vi "Teleop.vi"(10 "Match Info":T1={"Autonomous Elapsed Seconds"=0.0, "TeleOp Elapsed Seconds"=0.0, "Disabled Elapsed Seconds"=0.0, "Visited Autonomous"=FALSE, "Visited TeleOp"=FALSE, "Visited Disabled"=FALSE, "Autonomous Settings"={"Autonomous Style"=enum."Independent", "VI Refnum"=refnum}}, 11 "Call Context":T2) -> ()   [LabVIEW 2012]
doc: "This VI is called for each TeleOp packet received from the DS where the robot is not disabled. It is often used to read from the joysticks and update I/O or to update setpoints for timed control loops. It should complete and return within 20 milliseconds or it may miss DS packets."
uses:
  <vilib>/Rock Robotics/WPI/DriverStation/WPI_DriverStationDerivedRobotMode.ctl
  <vilib>/Rock Robotics/WPI/DriverStation/WPI_DriverStationMatch Info.ctl
  Global 1.vi
  Robot Global Data.vi
panel:
  in  "Boolean":bool
  in  "Percent":dbl
  out "RPM Number":dbl
  in  "RPM?":bool
  out "Actual RPM":dbl(slide) scale=0.0..4000.0
  in  "Input":dbl(slide) scale=0.0..1.0
  # "RPM"
  # "RPM"
  # "Power"
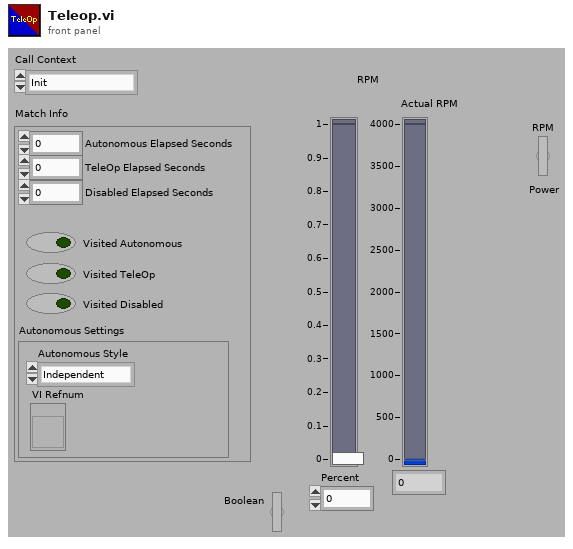
[diagram p1: front panel]
types:
  T1 = typedef "WPI_DriverStationMatch Info.ctl" = cluster{"Autonomous Elapsed Seconds":dbl, "TeleOp Elapsed Seconds":dbl, "Disabled Elapsed Seconds":dbl, "Visited Autonomous":bool, "Visited TeleOp":bool, "Visited Disabled":bool, "Autonomous Settings":cluster{"Autonomous Style":enum16{"Iterative", "Independent"}, "VI Refnum":refnum<vi>}}
  T2 = typedef "WPI_DriverStationDerivedRobotMode.ctl" = enum16{"Init", "Execute", "Stop"}
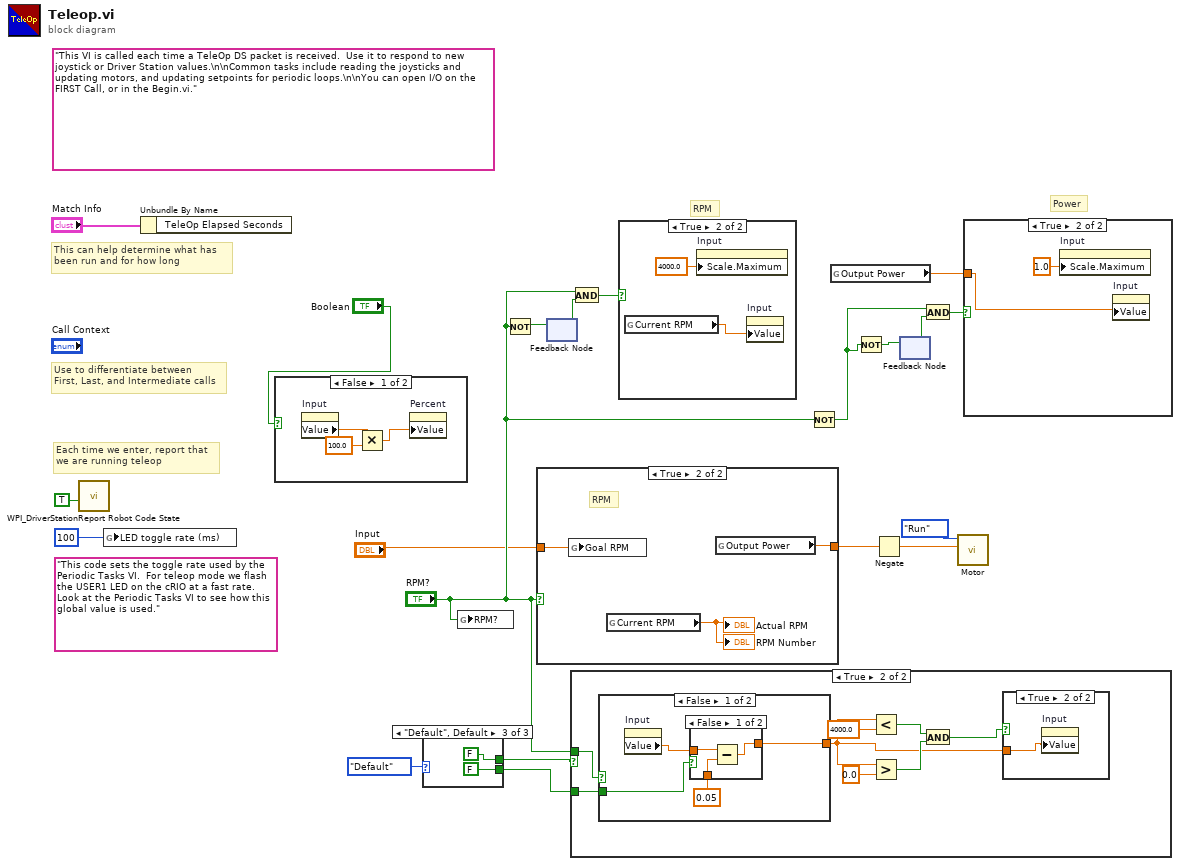
[diagram p0: block diagram]
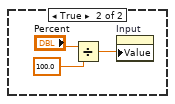
[diagram p2: hidden frame]
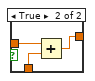
[diagram p5: hidden frame]
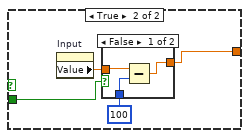
[diagram p6: hidden frame]
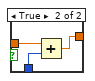
[diagram p7: hidden frame]
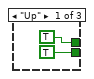
[diagram p8: hidden frame]
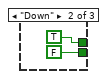
[diagram p9: hidden frame]
diagram:
  (unwired) "This code sets the toggle rate used by the Periodic Tasks VI.  For teleop mode we flash the USER1 LED on the cRIO at a fast rate.  Look at the Periodic Tasks VI to see how this global value is used."
  (unwired) "This VI is called each time a TeleOp DS packet is received.  Use it to respond to new joystick or Driver Station values.\n\nCommon tasks include reading the joysticks and updating motors, and updating setpoints for periodic loops.\n\nYou can open I/O on the FIRST Call, or in the Begin.vi."
  # "Power"
  # "RPM"
  # "Each time we enter, report that\nwe are running teleop"
  # "Use to differentiate between\nFirst, Last, and Intermediate calls"
  # "This can help determine what has\nbeen run and for how long"
  n1 = call <vilib>:"WPI_DriverStationReport Robot Code State.vi"("TeleOp"=TRUE ("Autonomous")) -> ()  [unwired: 10 in, 1 out]
  n2 = global write "Robot Global Data.vi" "LED toggle rate (ms)"(u32 100 ("LED ms toggle rate")) -> ()
  n3 = Unbundle By Name("Match Info") -> ()  [unwired: 1 out]
  n4 = case shown="False" "Boolean" {
    frame False {
      n5 = property on="Input" class="Slide (strict)"() -> ("Value"=w23:dbl)  [unwired: 2 in, 2 out]
      n6 = Multiply(x=w23, y=100.0) -> (x*y=w21:dbl)
      n7 = property on="Percent" class="DigNum (strict)"("Value"=w21) -> ()  [unwired: 2 in, 2 out]
    }
    frame True {
      n8 = Divide(x="Percent", y=100.0) -> (x/y=w24:dbl)
      n9 = property on="Input" class="Slide (strict)"("Value"=w24) -> ()  [unwired: 2 in, 2 out]
    }
  }
  n10 = case shown="\"Default\", Default" enum16{"Default", "Up", "Down"}."Default" {
    tunnel: [TRUE TRUE FALSE] -> w4
    tunnel: [TRUE FALSE FALSE] -> w10
    frame "Up" {
    }
    frame "Down" {
    }
    frame "Default", Default {
    }
  }
  n11 = global write "Global 1.vi" "RPM?"("RPM?") -> ()
  n12 = Not(x="RPM?") -> (.not. x?=w8:bool)
  n13 = case shown="True" "RPM?" {
    tunnel: [w33 w36] -> w11
    tunnel: "Input" -> [w33 w34]
    frame False {
      # "Power"
    }
    frame True {
      # "RPM"
      n14 = global write "Global 1.vi" "Goal RPM"(w34) -> ()
      n15 = global read "Global 1.vi" "Current RPM"() -> (→"Actual RPM" →"RPM Number":dbl)
      n16 = global read "Global 1.vi" "Output Power"() -> (w36:dbl)
    }
  }
  n17 = feedback-in #1(w8) -> ()
  n18 = feedback #1() -> (w16:bool)  [unwired: 1 in]
  n19 = case shown="True" w4 {
    tunnel: w10 -> [_ w44]
    tunnel: "RPM?" -> [_ w43]
    frame False {
    }
    frame True {
      n20 = case shown="False" w43 {
        tunnel: w44 -> [w47 w59]
        tunnel: [w46 w56] -> w37
        frame False {
          n21 = property on="Input" class="Slide (strict)"() -> ("Value"=w48:dbl)  [unwired: 2 in, 2 out]
          n22 = case shown="False" w47 {
            tunnel: w48 -> [w52 w55]
            tunnel: [w50 w54] -> w46
            tunnel: 0.05 -> [w51 w53]
            frame False {
              n23 = Subtract(x=w52, y=w51) -> (x-y=w50:dbl)
            }
            frame True {
              n24 = Add(x=w55, y=w53) -> (x+y=w54:dbl)
            }
          }
        }
        frame True {
          n25 = property on="Input" class="Slide (strict)"() -> ("Value"=w58:dbl)  [unwired: 2 in, 2 out]
          n26 = case shown="False" w59 {
            tunnel: w58 -> [w62 w65]
            tunnel: [w60 w64] -> w56
            tunnel: 100 -> [w61 w63]
            frame False {
              n27 = Subtract(x=w62, y=w61) -> (x-y=w60:dbl)
            }
            frame True {
              n28 = Add(x=w65, y=w63) -> (x+y=w64:dbl)
            }
          }
        }
      }
      n29 = Less?(x=w37, y=4000.0) -> (x < y?=w42:bool)
      n30 = Greater?(x=w37, y=0.0) -> (0:w38:bool)
      n31 = And(x=w42, y=w38) -> (x .and. y?=w41:bool)
      n32 = case shown="True" w41 {
        tunnel: w37 -> [_ w45]
        frame False {
        }
        frame True {
          n33 = property on="Input" class="Slide (strict)"("Value"=w45) -> ()  [unwired: 2 in, 2 out]
        }
      }
    }
  }
  n34 = And(x="RPM?", y=w16) -> (x .and. y?=w13:bool)
  n35 = case shown="True" w13 {
    frame False {
    }
    frame True {
      n36 = global read "Global 1.vi" "Current RPM"() -> (w66:dbl)
      n37 = property on="Input" class="Slide (strict)"("Scale.Maximum"=4000.0 ("Scale.Range:Maximum")) -> ()  [unwired: 2 in, 2 out]
      n38 = property on="Input" class="Slide (strict)"("Value"=w66) -> ()  [unwired: 2 in, 2 out]
    }
  }
  n39 = Not(x="RPM?") -> (.not. x?=w14:bool)
  n40 = global read "Global 1.vi" "Output Power"() -> (w6:dbl)
  n41 = Not(x=w14) -> (.not. x?=w7:bool)
  n42 = Negate(x=w11) -> (-x=w3:dbl)
  n43 = feedback #2() -> (w15:bool)  [unwired: 1 in]
  n44 = feedback-in #2(w7) -> ()
  n45 = And(x=w14, y=w15) -> (x .and. y?=w12:bool)
  n46 = call "Motor.vi"("Enum"=enum16{"Start", "Run", "End"}."Run", "Motor"=w3) -> ()  [unwired: 9 in]
  n47 = case shown="True" w12 {
    tunnel: w6 -> [_ w68]
    frame False {
    }
    frame True {
      n48 = property on="Input" class="Slide (strict)"("Scale.Maximum"=1.0 ("Scale.Range:Maximum")) -> ()  [unwired: 2 in, 2 out]
      n49 = property on="Input" class="Slide (strict)"("Value"=w68) -> ()  [unwired: 2 in, 2 out]
    }
  }
